vi "Create New Log File.vi"(8 "error in (no error)":errorcluster, 11 "Text File Sink in":refnum<class "Text File Sink.lvclass">) -> (0 "error out":errorcluster, 3 "Text File Sink out":refnum<class "Text File Sink.lvclass">)   [LabVIEW 2016, in "Stream Log.lvlib" / "Text File Sink.lvclass"]
doc: "--\nCopyright © 2017 Composed SystemsI All rights reserved.\n\nAuthor: Jon McBee <jon.mcbee@composed.io>\n\nThis library is provided \"AS IS\" ,WITHOUT WARRANTIES OR\nCONDITIONS OF ANY KIND, either express or implied.\n\nComposed Systems -- composed.io\n\nStream 0.0.1.1\nJon McBee - Composed Systems\nCopyright (c) 2017, Composed Systems"
uses:
  <userlib>/Composed Systems/Stream/Log/Text File Sink/Text File Sink.lvclass
  <userlib>/Composed Systems/Stream/Log/Text File Sink/Text File Sink.lvclass/Text File Sink.ctl
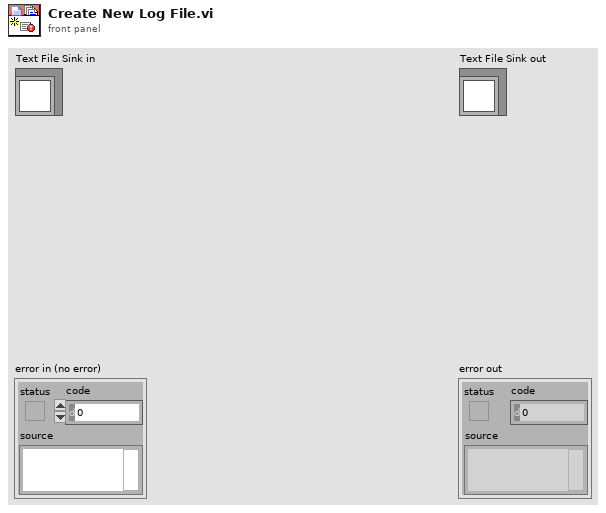
[diagram p1: front panel]
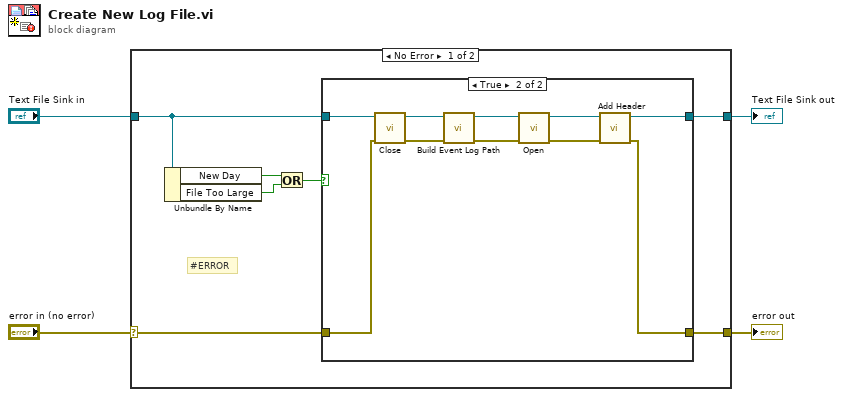
[diagram p0: block diagram]
diagram:
  n1 = case shown="No Error" "error in (no error)" {
    selector: "error in (no error)" -> [w6 w25]
    tunnel: [w5 w25] -> w3
    tunnel: [w7 w24] -> w1
    tunnel: "Text File Sink in" -> [w8 w24]
    frame No Error {
      # "#ERROR"
      n2 = Unbundle By Name(w8) -> ("New Day"=w11:bool, "File Too Large"=w10:bool)
      n3 = Or(x=w11, y=w10) -> (x .or. y?=w9:bool)
      n4 = case shown="True" w9 {
        tunnel: w8 -> [w12 w23]
        tunnel: [w12 w19] -> w7
        tunnel: [w13 w14] -> w5
        tunnel: w6 -> [w13 w15]
        frame False {
        }
        frame True {
          n5 = call <userlib>:"Close.vi"("error in (no error)"=w15, "Text File Sink in"=w23) -> ("error out"=w18:errorcluster, "Text File Sink out"=w22:refnum<class "Text File Sink.lvclass">)  [unwired: 8 in]
          n6 = call <userlib>:"Build Event Log Path.vi"("error in (no error)"=w18, "Text File Sink in"=w22) -> ("error out"=w17:errorcluster, "Text File Sink out"=w21:refnum<class "Text File Sink.lvclass">)  [unwired: 8 in]
          n7 = call <userlib>:"Open.vi"("error in (no error)"=w17, "Text File Sink in"=w21) -> ("error out"=w16:errorcluster, "Text File Sink out"=w20:refnum<class "Text File Sink.lvclass">)  [unwired: 8 in]
          n8 = call-dynamic "Add Header.vi"("error in (no error)"=w16, "Text File Sink in"=w20) -> ("error out"=w14:errorcluster, "Text File Sink out"=w19:refnum<class "Text File Sink.lvclass">)  [unwired: 8 in]
        }
      }
    }
    frame Error {
    }
  }
  "error out" <- w3
  "Text File Sink out" <- w1
